vi "ZeitabhängigeTXTerstellen.vi"(10 "Kanal":string, 11 "path":path) -> (3 "Path":path)   [LabVIEW 2023]
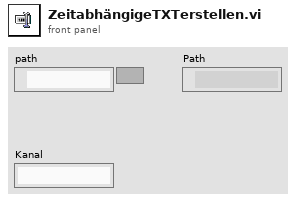
[diagram p1: front panel]
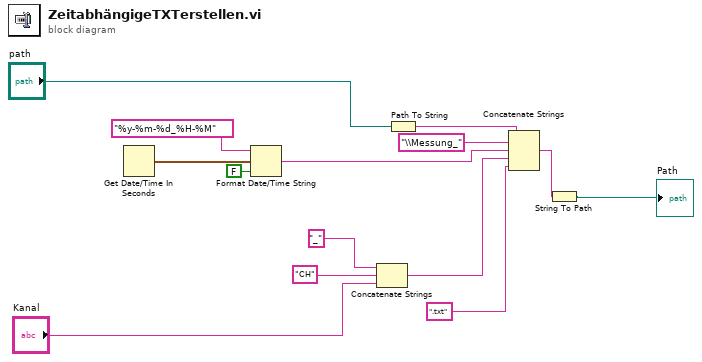
[diagram p0: block diagram]
diagram:
  n1 = Get Date/Time In Seconds() -> (seconds since 1Jan1904=w9:timestamp)
  n2 = Format Date/Time String(time format string (%c)="%y-%m-%d_%H-%M", seconds (now)=w9, UTC format=FALSE) -> (date/time string=w10:string)
  n3 = Concatenate Strings("_" ("string"), "CH" ("string"), "Kanal") -> (w11:string)
  n4 = Path To String(path="path") -> (string=w3:string)
  n5 = Concatenate Strings(w3, "\\Messung_" ("string"), w10, w11, ".txt" ("element")) -> (w4:string)
  n6 = String To Path(string=w4) -> (path=→"Path":path)
